vi "Database Name and Path.vi"(8 "error in (no error)":errorcluster) -> (0 "error out":errorcluster, 2 "database name":string, 3 "databse path":path)   [LabVIEW 2018, in "Dynamic Shared Variables.lvlib"]
doc: "Returns the name and path of the database. If the folder does not exist, it creates it."
uses:
  Dynamic Shared Variables.lvlib
  <vilib>/Utility/sysdir.llb/System Directory Type.ctl
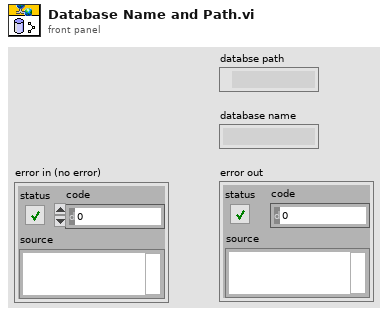
[diagram p1: front panel]
types:
  T1 = typedef "System Directory Type.ctl" = i32
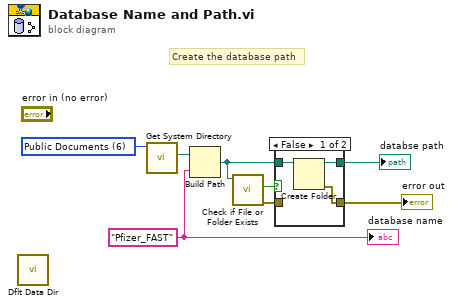
[diagram p0: block diagram]
diagram:
  w8 = "Pfizer_FAST" ("name or relative path")
  w6 = T1 6 items=["User Home"=0, "User Desktop"=1, "User Documents"=2, "User Application Data"=3, "User Preferences"=4, "User Temporary"=5, "Public Documents"=6, "Public Application Data"=7, "Public Preferences"=8, "Public Cache"=13, "System Core Libraries"=9, "System Installed Libraries"=10, "Application Files"=11, "Boot Volume Root"=12] ("system directory type")
  # "Create the database path"
  n1 = call <vilib>:"Dflt Data Dir.vi"() -> ()  [unwired: 1 out]
  n2 = call <vilib>:"Get System Directory.vi"("system directory type"=w6) -> ("system directory"=w7:path)  [unwired: 10 in]
  n3 = Build Path(base path=w7, name or relative path=w8) -> (appended path=w1:path)
  n4 = call <vilib>:"Check if File or Folder Exists.vi"("path"=w1) -> ("error out"=w4:errorcluster, "file or folder exists?"=w2:bool)  [unwired: 8 in, 1 out]
  n5 = case shown="False" w2 {
    tunnel: w1 -> [w11 w12]
    tunnel: [w10 w13] -> w3
    tunnel: w4 -> [_ w13]
    tunnel: [w9 w12] -> w5
    frame False {
      n6 = Create Folder(path (use dialog)=w11) -> (created path=w9:path, error out=w10:errorcluster)  [unwired: 2 in, 1 out]
    }
    frame True {
    }
  }
  "databse path" <- w5
  "error out" <- w3
  "database name" <- w8
